vi "TimingEstimate_Valid_Invalid_Update.vi"(7 "Command":enum16{"Valid", "Invalid"}(ring), 8 "error in (no error)":errorcluster, 11 "UI control refnums":T1) -> (0 "error out":errorcluster)   [LabVIEW 2012]
doc: "SciScan 1.2 160622"
uses:
  Custom Controls and Typedefs/Macro_MD_UI Control Refnums.ctl
  Custom Controls and Typedefs/Delete Button.ctl
  Custom Controls and Typedefs/Edit Button.ctl
  Custom Controls and Typedefs/Timing Estimate Cluster.ctl
  CommonResource VIs/Timing/Timing Indicator.ctl
  Custom Controls and Typedefs/Load from PSM Button.ctl
panel:
  # "(hh:mm:ss)"
  # "(hh:mm:ss)"
  # "(hh:mm:ss)"
  # "(hh:mm:ss)"
  # "(hh:mm:ss)"
  # "(hh:mm:ss)"
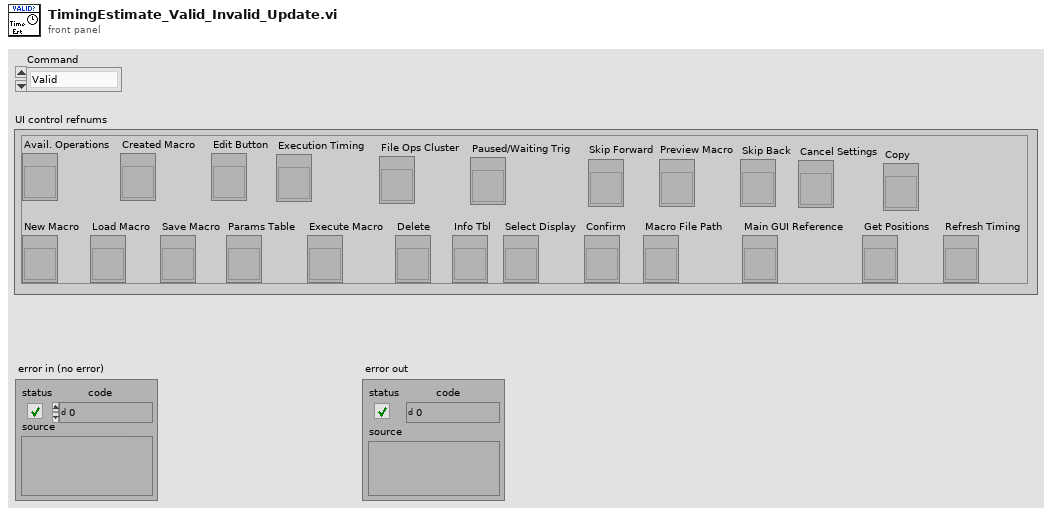
[diagram p1: front panel]
types:
  T1 = typedef "Macro_MD_UI Control Refnums.ctl" = cluster{"Avail. Operations":refnum<vi>, "Created Macro":refnum<vi>, "Load Macro":refnum<vi>, "Save Macro":refnum<vi>, "Params Table":refnum<vi>, "Delete":refnum<vi>, "Edit Button":refnum<vi>, "Execute Macro":refnum<vi>, "Info Tbl":refnum<vi>, "Execution Timing":refnum<vi>, "Select Display":refnum<vi>, "File Ops Cluster":refnum<vi>, "Paused/Waiting Trig":refnum<vi>, "Confirm":refnum<vi>, "New Macro":refnum<vi>, "Preview Macro":refnum<vi>, "Skip Forward":refnum<vi>, "Skip Back":refnum<vi>, "Macro File Path":refnum<vi>, "Main GUI Reference":refnum<vi>, "Cancel Settings":refnum<vi>, "Get Positions":refnum<vi>, "Copy":refnum<vi>, "Refresh Timing":refnum<vi>}
  T2 = typedef "Timing Estimate Cluster.ctl" = cluster{"Est. Time":dbl, "Remaining":dbl, "Progress":u8, "Elapsed":dbl}
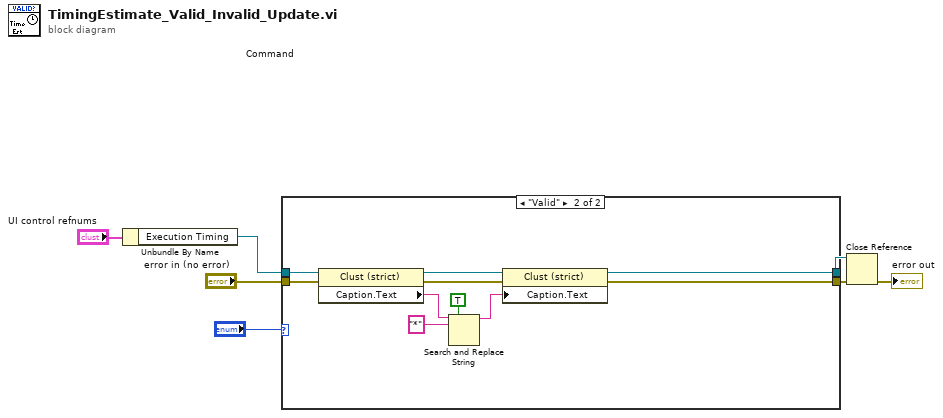
[diagram p0: block diagram]
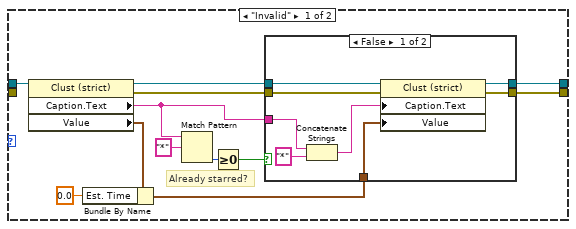
[diagram p2: hidden frame]
diagram:
  n1 = Unbundle By Name("UI control refnums") -> ("Execution Timing"=w5:refnum<vi>)
  n2 = case shown="\"Valid\"" "Command" {
    tunnel: w5 -> [w19 w39]
    tunnel: "error in (no error)" -> [_ w36]
    tunnel: [w9 w35] -> w3
    tunnel: [w8 w34] -> w2
    frame "Invalid" {
      # "Already starred?"
      n3 = property class="Clust (strict)"(reference=w19) -> (reference out=w11:refnum<vi>, error out=w12:errorcluster, "Caption.Text"=w15:string, "Value"=w18:T2)  [unwired: 1 in]
      n4 = Bundle By Name(cluster=w18, "Est. Time"=0.0) -> (w10:T2)
      n5 = Match Pattern(string=w15, regular expression="*") -> (offset past match=w14:i32)  [unwired: 1 in, 3 out]
      n6 = Greater Or Equal To 0?(x=w14) -> (x >= 0?=w13:bool)
      n7 = case shown="False" w13 {
        tunnel: w15 -> [w27 _]
        tunnel: w12 -> [w24 w29]
        tunnel: w11 -> [w23 w28]
        tunnel: w10 -> [w22 _]
        tunnel: [w21 w29] -> w9
        tunnel: [w20 w28] -> w8
        frame False {
          n8 = Concatenate Strings(w27, "*" ("string")) -> (w25:string)
          n9 = property class="Clust (strict)"(reference=w23, error in=w24, "Caption.Text"=w25, "Value"=w22) -> (reference out=w20:refnum<vi>, error out=w21:errorcluster)
        }
        frame True {
        }
      }
    }
    frame "Valid" {
      n10 = property class="Clust (strict)"(reference=w39, error in=w36) -> (reference out=w38:refnum<vi>, error out=w37:errorcluster, "Caption.Text"=w33:string)
      n11 = Search and Replace String(replace all?=TRUE ("replace all? (F)"), input string=w33, search string="*") -> (result string=w31:string)  [unwired: 5 in, 3 out]
      n12 = property class="Clust (strict)"(reference=w38, error in=w37, "Caption.Text"=w31) -> (reference out=w34:refnum<vi>, error out=w35:errorcluster)
    }
  }
  n13 = Close Reference(reference=w2, error in (no error)=w3) -> (error out=→"error out":errorcluster)
